vi "Measure.vi"(8 "error in (no error)":errorcluster, 9 "measurement configuration":variant, 10 "measure call context in":refnum<class "Measure Call Context.lvclass">, 11 "measurement plugin in":refnum<class "Workflow DO.lvclass">) -> (0 "error out":errorcluster, 1 "measurement results":variant, 2 "measure call context out":refnum<class "Measure Call Context.lvclass">, 3 "measurement plugin out":refnum<class "Workflow DO.lvclass">)   [LabVIEW 2025, in "Workflow DO.lvclass"]
uses:
  Workflow DO.lvclass
  <vilib>/Plug-In SDKs/Measurements/Measure Call Context/Measure Call Context.lvclass
  Measurement Configuration.ctl
  Workflow DO.lvclass/Workflow DO.ctl
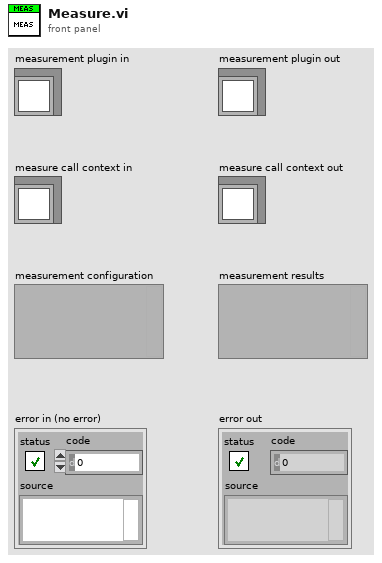
[diagram p1: front panel]
types:
  T1 = typedef "Workflow DO.lvclass/Measurement Configuration.ctl" = cluster{"Input Terminal Name":string, "Counter Interface":string, "Active Edge":i32, "Pulses":u32, "Timeout (s)":u32, "FD Baudrate":u32, "Baudrate":u32, "FD ISO Mode":enum32{"ISO", "Legacy ISO", "Non-ISO"}, "IO Mode":enum32{"CAN", "CAN FD", "CAN FD + BRS"}, "Can Interface":string, "Termination CAN":bool, "IDENTIFIER":u32, "PAYLOAD":u32[]}
  T2 = typedef "Workflow DO.lvclass/Measurement Results.ctl" = cluster{"Count":u32}
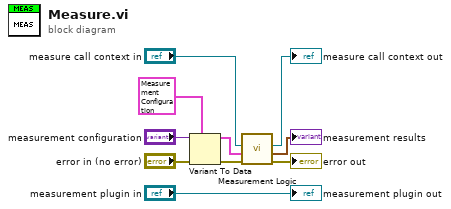
[diagram p0: block diagram]
diagram:
  n1 = Variant To Data(error in="error in (no error)", type=T1 {"Input Terminal Name"="Lorem ipsum dolor sit", "Counter Interface"="", "Active Edge"=1, "Pulses"=32, "Timeout (s)"=64, "FD Baudrate"=4294967264, "Baudrate"=4294967264, "FD ISO Mode"=enum."ISO", "IO Mode"=enum."CAN", "Can Interface"="", "Termination CAN"=TRUE, "IDENTIFIER"=1, "PAYLOAD"=[3, 6]} ("measurement configuration"), Variant="measurement configuration") -> (data=w1:T1, error out=w7:errorcluster)
  n2 = call "Measurement Logic.vi"("error in"=w7, "measurement configuration"=w1, "measure call context in"="measure call context in") -> ("error out"=→"error out":errorcluster, "measurement results"=→"measurement results":T2, "measure call context out"=→"measure call context out":refnum<class "Measure Call Context.lvclass">)  [unwired: 6 in]
  "measurement plugin out" <- "measurement plugin in"
